vi "Series Recognition.vi"(8 "error in (no error)":errorcluster, 10 "Series Type (0: MXG)":u16(ring) items=["MXG", "PSG", "PSG-A", "PSG-C", "PSG-D"], 11 "VISA resource name":refnum<visa-resource-name>) -> (0 "error out":errorcluster, 2 "Is Series Correct":bool, 3 "VISA resource name out":refnum<visa-resource-name>)   [LabVIEW 2011, in "Agilent PSG MXG Series.lvlib"]
doc: "Specifies whether the series is correct."
uses:
  Agilent PSG MXG Series.lvlib
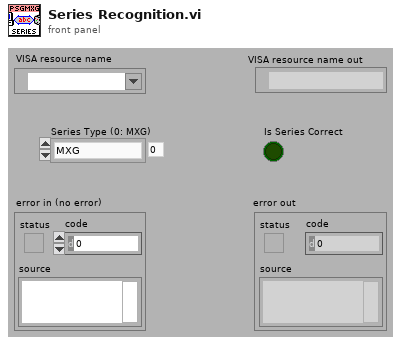
[diagram p1: front panel]
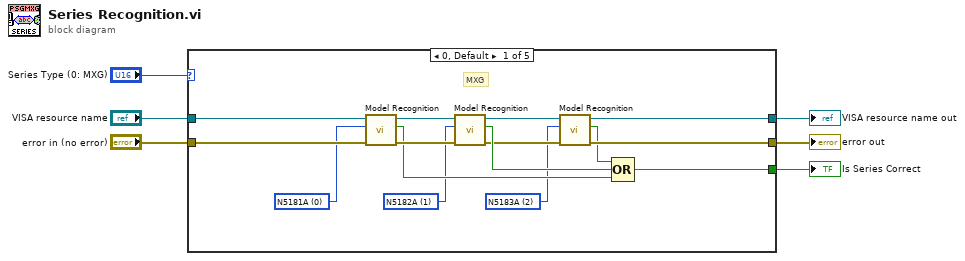
[diagram p0: block diagram]
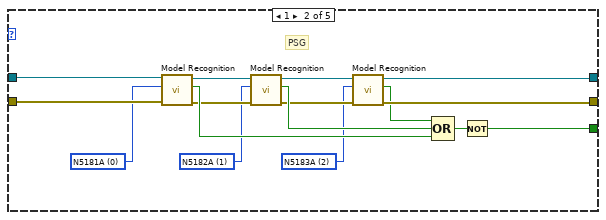
[diagram p2: hidden frame]
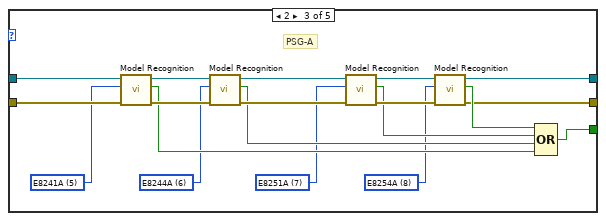
[diagram p3: hidden frame]
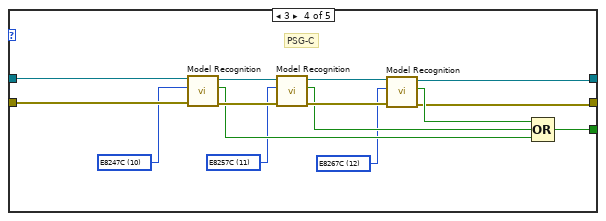
[diagram p4: hidden frame]
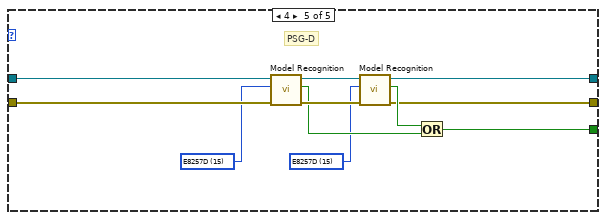
[diagram p5: hidden frame]
diagram:
  n1 = case shown="0, Default" "Series Type (0: MXG)" {
    tunnel: "VISA resource name" -> [w21 w33 w54 w69 w78]
    tunnel: "error in (no error)" -> [w20 w32 w53 w62 w77]
    tunnel: [w15 w28 w44 w63 w76] -> w3
    tunnel: [w10 w25 w43 w61 w75] -> w2
    tunnel: [w9 w24 w42 w60 w74] -> w1
    frame 0, Default {
      w8 = u16 2 items=["N5181A"=0, "N5182A"=1, "N5183A"=2, "E8241A"=5, "E8244A"=6, "E8251A"=7, "E8254A"=8, "E8247C"=10, "E8257C"=11, "E8267C"=12, "E8257D"=15, "E8267D"=16] ("Model Type (0: N5181A)")
      w13 = u16 1 items=["N5181A"=0, "N5182A"=1, "E8241A"=5, "E8244A"=6, "E8251A"=7, "E8254A"=8, "E8247C"=10, "E8257C"=11, "E8267C"=12, "E8257D"=15, "E8267D"=16] ("Model Type (0: N5181A)")
      w14 = u16 0 items=["N5181A"=0, "N5182A"=1, "E8241A"=5, "E8244A"=6, "E8251A"=7, "E8254A"=8, "E8247C"=10, "E8257C"=11, "E8267C"=12, "E8257D"=15, "E8267D"=16] ("Model Type (0: N5181A)")
      # "MXG"
      n2 = call "Model Recognition.vi"("error in (no error)"=w20, "Model Type (0: N5181A)"=w14, "VISA resource name"=w21) -> ("error out"=w18:errorcluster, "Is Model Correct"=w17:bool, "VISA resource name out"=w19:refnum<visa-resource-name>)  [unwired: 6 in]
      n3 = call "Model Recognition.vi"("error in (no error)"=w18, "Model Type (0: N5181A)"=w13, "VISA resource name"=w19) -> ("error out"=w11:errorcluster, "Is Model Correct"=w16:bool, "VISA resource name out"=w12:refnum<visa-resource-name>)  [unwired: 6 in]
      n4 = call "Model Recognition.vi"("error in (no error)"=w11, "Model Type (0: N5181A)"=w8, "VISA resource name"=w12) -> ("error out"=w9:errorcluster, "Is Model Correct"=w7:bool, "VISA resource name out"=w10:refnum<visa-resource-name>)  [unwired: 6 in]
      n5 = Compound Arithmetic op=OR(w7, w16, w17) -> (w15:bool)
    }
    frame 1 {
      w23 = u16 2 items=["N5181A"=0, "N5182A"=1, "N5183A"=2, "E8241A"=5, "E8244A"=6, "E8251A"=7, "E8254A"=8, "E8247C"=10, "E8257C"=11, "E8267C"=12, "E8257D"=15, "E8267D"=16] ("Model Type (0: N5181A)")
      w30 = u16 1 items=["N5181A"=0, "N5182A"=1, "E8241A"=5, "E8244A"=6, "E8251A"=7, "E8254A"=8, "E8247C"=10, "E8257C"=11, "E8267C"=12, "E8257D"=15, "E8267D"=16] ("Model Type (0: N5181A)")
      w31 = u16 0 items=["N5181A"=0, "N5182A"=1, "E8241A"=5, "E8244A"=6, "E8251A"=7, "E8254A"=8, "E8247C"=10, "E8257C"=11, "E8267C"=12, "E8257D"=15, "E8267D"=16] ("Model Type (0: N5181A)")
      # "PSG"
      n6 = call "Model Recognition.vi"("error in (no error)"=w32, "Model Type (0: N5181A)"=w31, "VISA resource name"=w33) -> ("error out"=w35:errorcluster, "Is Model Correct"=w36:bool, "VISA resource name out"=w34:refnum<visa-resource-name>)  [unwired: 6 in]
      n7 = call "Model Recognition.vi"("error in (no error)"=w35, "Model Type (0: N5181A)"=w30, "VISA resource name"=w34) -> ("error out"=w26:errorcluster, "Is Model Correct"=w37:bool, "VISA resource name out"=w27:refnum<visa-resource-name>)  [unwired: 6 in]
      n8 = call "Model Recognition.vi"("error in (no error)"=w26, "Model Type (0: N5181A)"=w23, "VISA resource name"=w27) -> ("error out"=w24:errorcluster, "Is Model Correct"=w22:bool, "VISA resource name out"=w25:refnum<visa-resource-name>)  [unwired: 6 in]
      n9 = Compound Arithmetic op=OR(w22, w37, w36) -> (w29:bool)
      n10 = Not(x=w29) -> (.not. x?=w28:bool)
    }
    frame 2 {
      w38 = u16 8 items=["N5181A"=0, "N5182A"=1, "E8241A"=5, "E8244A"=6, "E8251A"=7, "E8254A"=8, "E8247C"=10, "E8257C"=11, "E8267C"=12, "E8257D"=15, "E8267D"=16] ("Model Type (0: N5181A)")
      w39 = u16 7 items=["N5181A"=0, "N5182A"=1, "E8241A"=5, "E8244A"=6, "E8251A"=7, "E8254A"=8, "E8247C"=10, "E8257C"=11, "E8267C"=12, "E8257D"=15, "E8267D"=16] ("Model Type (0: N5181A)")
      w40 = u16 6 items=["N5181A"=0, "N5182A"=1, "E8241A"=5, "E8244A"=6, "E8251A"=7, "E8254A"=8, "E8247C"=10, "E8257C"=11, "E8267C"=12, "E8257D"=15, "E8267D"=16] ("Model Type (0: N5181A)")
      w41 = u16 5 items=["N5181A"=0, "N5182A"=1, "E8241A"=5, "E8244A"=6, "E8251A"=7, "E8254A"=8, "E8247C"=10, "E8257C"=11, "E8267C"=12, "E8257D"=15, "E8267D"=16] ("Model Type (0: N5181A)")
      # "PSG-A"
      n11 = call "Model Recognition.vi"("error in (no error)"=w53, "Model Type (0: N5181A)"=w41, "VISA resource name"=w54) -> ("error out"=w56:errorcluster, "Is Model Correct"=w48:bool, "VISA resource name out"=w55:refnum<visa-resource-name>)  [unwired: 6 in]
      n12 = call "Model Recognition.vi"("error in (no error)"=w56, "Model Type (0: N5181A)"=w40, "VISA resource name"=w55) -> ("error out"=w49:errorcluster, "Is Model Correct"=w47:bool, "VISA resource name out"=w50:refnum<visa-resource-name>)  [unwired: 6 in]
      n13 = call "Model Recognition.vi"("error in (no error)"=w49, "Model Type (0: N5181A)"=w39, "VISA resource name"=w50) -> ("error out"=w52:errorcluster, "Is Model Correct"=w46:bool, "VISA resource name out"=w51:refnum<visa-resource-name>)  [unwired: 6 in]
      n14 = call "Model Recognition.vi"("error in (no error)"=w52, "Model Type (0: N5181A)"=w38, "VISA resource name"=w51) -> ("error out"=w42:errorcluster, "Is Model Correct"=w45:bool, "VISA resource name out"=w43:refnum<visa-resource-name>)  [unwired: 6 in]
      n15 = Compound Arithmetic op=OR(w45, w46, w47, w48) -> (w44:bool)
    }
    frame 3 {
      w57 = u16 12 items=["N5181A"=0, "N5182A"=1, "E8241A"=5, "E8244A"=6, "E8251A"=7, "E8254A"=8, "E8247C"=10, "E8257C"=11, "E8267C"=12, "E8257D"=15, "E8267D"=16] ("Model Type (0: N5181A)")
      w58 = u16 11 items=["N5181A"=0, "N5182A"=1, "E8241A"=5, "E8244A"=6, "E8251A"=7, "E8254A"=8, "E8247C"=10, "E8257C"=11, "E8267C"=12, "E8257D"=15, "E8267D"=16] ("Model Type (0: N5181A)")
      w59 = u16 10 items=["N5181A"=0, "N5182A"=1, "E8241A"=5, "E8244A"=6, "E8251A"=7, "E8254A"=8, "E8247C"=10, "E8257C"=11, "E8267C"=12, "E8257D"=15, "E8267D"=16] ("Model Type (0: N5181A)")
      # "PSG-C"
      n16 = call "Model Recognition.vi"("error in (no error)"=w62, "Model Type (0: N5181A)"=w59, "VISA resource name"=w69) -> ("error out"=w71:errorcluster, "Is Model Correct"=w66:bool, "VISA resource name out"=w70:refnum<visa-resource-name>)  [unwired: 6 in]
      n17 = call "Model Recognition.vi"("error in (no error)"=w71, "Model Type (0: N5181A)"=w58, "VISA resource name"=w70) -> ("error out"=w67:errorcluster, "Is Model Correct"=w65:bool, "VISA resource name out"=w68:refnum<visa-resource-name>)  [unwired: 6 in]
      n18 = call "Model Recognition.vi"("error in (no error)"=w67, "Model Type (0: N5181A)"=w57, "VISA resource name"=w68) -> ("error out"=w60:errorcluster, "Is Model Correct"=w64:bool, "VISA resource name out"=w61:refnum<visa-resource-name>)  [unwired: 6 in]
      n19 = Compound Arithmetic op=OR(w64, w65, w66) -> (w63:bool)
    }
    frame 4 {
      w72 = u16 15 items=["N5181A"=0, "N5182A"=1, "E8241A"=5, "E8244A"=6, "E8251A"=7, "E8254A"=8, "E8247C"=10, "E8257C"=11, "E8267C"=12, "E8257D"=15, "E8267D"=16] ("Model Type (0: N5181A)")
      w73 = u16 15 items=["N5181A"=0, "N5182A"=1, "E8241A"=5, "E8244A"=6, "E8251A"=7, "E8254A"=8, "E8247C"=10, "E8257C"=11, "E8267C"=12, "E8257D"=15, "E8267D"=16] ("Model Type (0: N5181A)")
      # "PSG-D"
      n20 = call "Model Recognition.vi"("error in (no error)"=w77, "Model Type (0: N5181A)"=w73, "VISA resource name"=w78) -> ("error out"=w81:errorcluster, "Is Model Correct"=w80:bool, "VISA resource name out"=w82:refnum<visa-resource-name>)  [unwired: 6 in]
      n21 = call "Model Recognition.vi"("error in (no error)"=w81, "Model Type (0: N5181A)"=w72, "VISA resource name"=w82) -> ("error out"=w74:errorcluster, "Is Model Correct"=w79:bool, "VISA resource name out"=w75:refnum<visa-resource-name>)  [unwired: 6 in]
      n22 = Or(x=w79, y=w80) -> (x .or. y?=w76:bool)
    }
  }
  "error out" <- w1
  "VISA resource name out" <- w2
  "Is Series Correct" <- w3
